vi "Ultrasonic.vi"(1 "Right":T1=enum."AI 2", 2 "State Control":enum16{"Open", "Run", "End"}(ring)) -> ()   [LabVIEW 2013]
doc: "This example shows how to use the MaxBotix LV-MaxSonar-EZ1 Sonar Range Finder MB1010. It will display the distance from the sensor in inches.\n\nThis example works with the NI 9201 module with an Analog Breakout attached. The Analog Breakout should have 12V applied to the WAGO connector (J3). The sensor is attached to the 3x8 header using a 3-pin PWM connector."
uses:
  <vilib>/Rock Robotics/SystemInterfaces/AI/FPGA_AIChannel.ctl
panel:
  out "Left distance":dbl(slide)=125.0 scale=0.0..250.0 scale format="%3d"
  out "Left Distance":dbl
  out "Left Waveform":dbl(graph)
  out "Right Distance":dbl
  out "Right Waveform Chart":dbl(graph)
  out "Right distance":dbl(slide)=125.0 scale=0.0..250.0 scale format="%3d"
  in  "Left":T1
  # "Set these inputs before running."
  # "Wiring Diagram for Analog Breakout connected to an NI 9201"
  # "EZ1 MB1010"
  # "This shows wiring for a MaxBotix LV-MaxSonar-EZ1 Sonar Range Finder MB1010."
  # "GND"
  # "+5"
  # "TX"
  # "RX"
  # "AN"
  # "PW"
  # "BW"
  # "jumper to read battery or AI8"
  # "GND"
  # "SIG"
  # "5V"
  # "AI8\nAI7\nAI6\nAI5\nAI4\nAI3\nAI2\nAI1"
  # "+"
  # "12V from battery"
  # "-"
  # "\"power good\" LED"
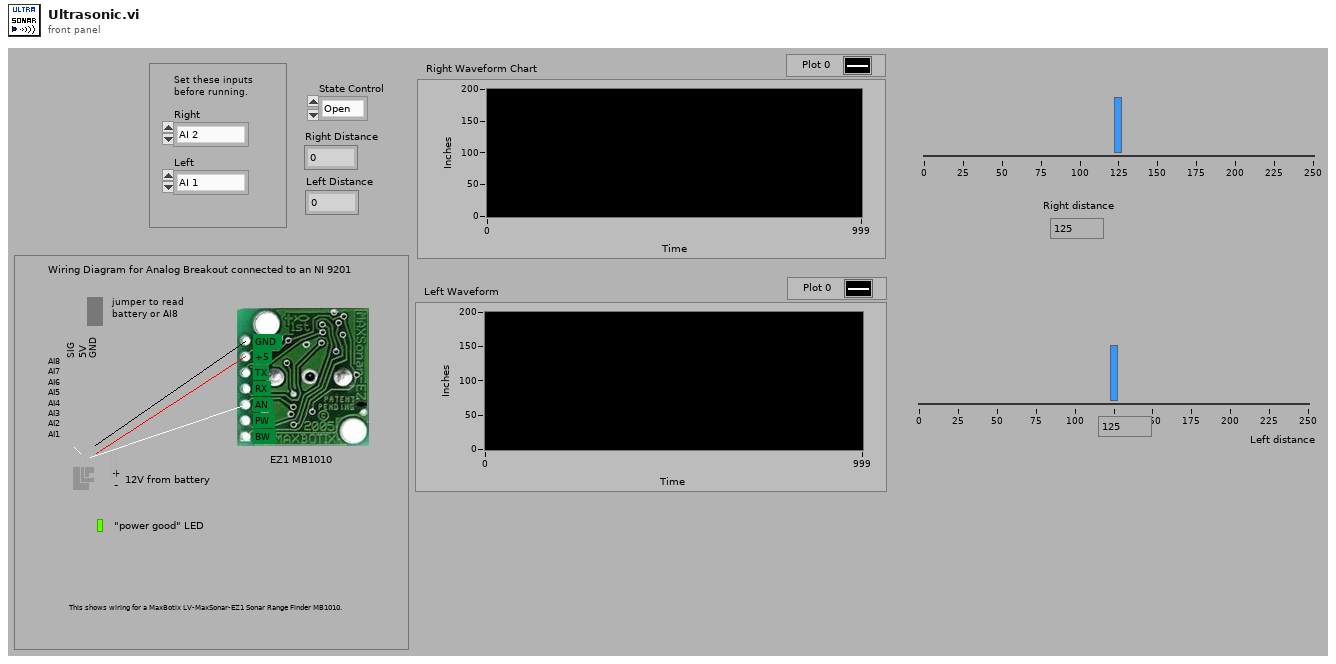
[diagram p1: front panel]
types:
  T1 = typedef "FPGA_AIChannel.ctl" = enum8{"AI 1", "AI 2", "AI 3", "AI 4", "AI 5", "AI 6", "AI 7", "AI 8", "Invalid"}
  T2 = typedef "WPI_AnalogChannelDevRef.ctl" = cluster{"DevStatus":errorcluster, "Analog Module":T3, "Analog Channel":T1}
  T3 = typedef "FPGA_TypedefAnalogModule.ctl" = enum16{"Analog Module 1", "Analog Module 2"}
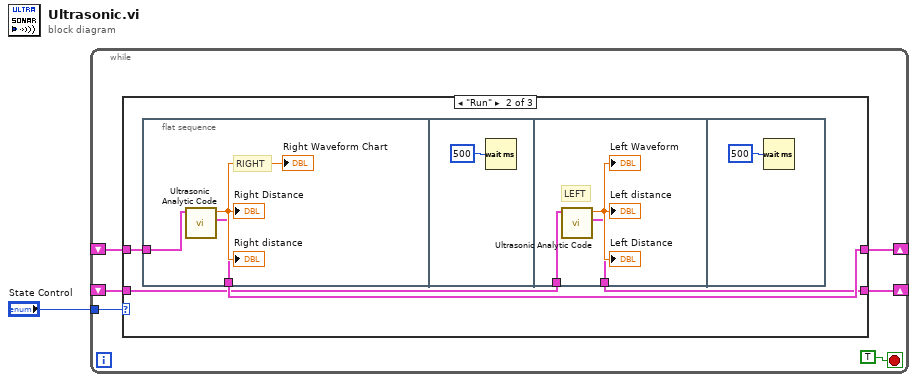
[diagram p0: block diagram]
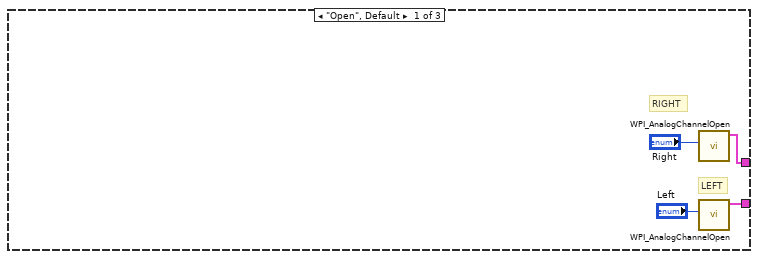
[diagram p2: hidden frame]
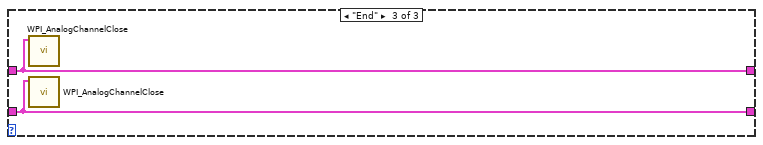
[diagram p3: hidden frame]
diagram:
  n1 = while {
    tunnel: "State Control" -> [w7]
    shift-right: [w6] -> _
    shift-left: _ -> [w5]
    shift-right: [w3] -> _
    shift-left: _ -> [w2]
    stop <- TRUE stop-if-true
    n2 = case shown="\"Run\"" w7 {
      tunnel: [w10 w14 w25] -> w6
      tunnel: w5 -> [_ w15 w25]
      tunnel: [w8 w12 w24] -> w3
      tunnel: w2 -> [_ w13 w24]
      frame "Open", Default {
        # "LEFT"
        # "RIGHT"
        n3 = call <vilib>:"WPI_AnalogChannelOpen.vi"("Analog Channel"="Right") -> ("AIDeviceRef"=w10:T2)  [unwired: 2 in, 8 out]
        n4 = call <vilib>:"WPI_AnalogChannelOpen.vi"("Analog Channel"="Left") -> ("AIDeviceRef"=w8:T2)  [unwired: 2 in, 8 out]
      }
      frame "Run" {
        n5 = flat-sequence {
          tunnel: w15 -> [w17]
          tunnel: [w16] -> w14
          tunnel: w13 -> [w21]
          tunnel: [w20] -> w12
          frame #0 {
            # "RIGHT"
            n6 = call "Ultrasonic Analytic Code.vi"("AIDeviceRef 2"=w17) -> ("AIDeviceRef"=w16:T2, "Distance"=→"Right distance" →"Right Waveform Chart" →"Right Distance":dbl)  [unwired: 9 in]
          }
          frame #1 {
            n7 = Wait (ms)(milliseconds to wait=u32 500) -> ()  [unwired: 1 out]
          }
          frame #2 {
            # "LEFT"
            n8 = call "Ultrasonic Analytic Code.vi"("AIDeviceRef 2"=w21) -> ("AIDeviceRef"=w20:T2, "Distance"=→"Left Waveform" →"Left Distance" →"Left distance":dbl)  [unwired: 9 in]
          }
          frame #3 {
            n9 = Wait (ms)(milliseconds to wait=u32 500) -> ()  [unwired: 1 out]
          }
        }
      }
      frame "End" {
        n10 = call <vilib>:"WPI_AnalogChannelClose.vi"("AIDeviceRef"=w25) -> ()  [unwired: 1 in, 10 out]
        n11 = call <vilib>:"WPI_AnalogChannelClose.vi"("AIDeviceRef"=w24) -> ()  [unwired: 1 in, 10 out]
      }
    }
  }
